vi "pmu_Check Channel Error (Std 2011).vi"(8 "error in (no error)":errorcluster, 10 "physical channel in":T3(array[cluster]), 11 "phasor channels":T4[](array[typedef]) {"phasor unit scaling" max=16777215 format="%06x"; "phasor unit" items=["Voltage [V]"=0, "Current [A]"=16777216]}) -> (0 "error out":errorcluster, 3 "phasor channel info":T1[](array[typedef]))   [LabVIEW 2014, in "NI_EP_PMU.lvlib"]
uses:
  <vilib>/addons/Electrical Power/PMU/NI_EP_PMU.lvlib
  <vilib>/addons/Electrical Power/PMU/Common/Controls/pmu_Phasor Channel.ctl
  <vilib>/addons/Electrical Power/PMU/Common/Controls/pmu_Channel Phase.ctl
  <vilib>/addons/Electrical Power/PMU/Common/Controls/pmu_Phasor Channel Info.ctl
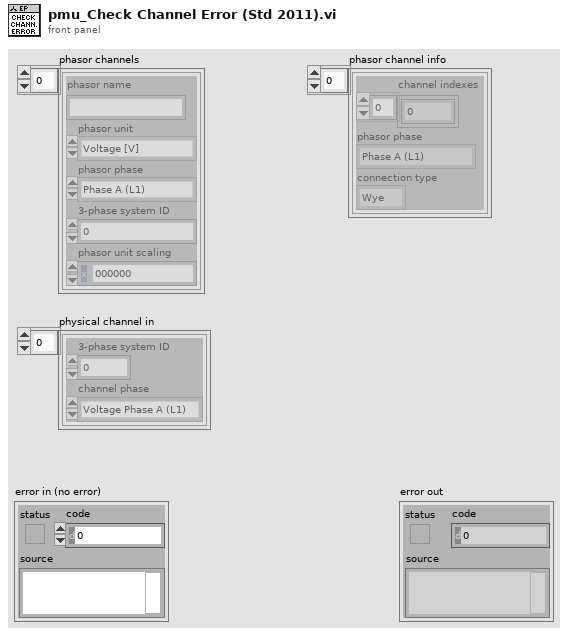
[diagram p1: front panel]
types:
  T1 = typedef "NI_EP_PMU.lvlib/pmu_Phasor Channel Info.ctl" = cluster{"channel indexes":i32[], "phasor phase":enum16{"Phase A (L1)", "Phase B (L2)", "Phase C (L3)", "Phase N", "Positive sequence", "Negative sequence", "Zero sequence"}, "connection type":enum16{"Wye", "Delta"}}
  T2 = typedef "NI_EP_PMU.lvlib/pmu_Channel Phase.ctl" = enum16{"Voltage Phase A (L1)", "Voltage Phase B (L2)", "Voltage Phase C (L3)", "Voltage Phase N (Neutral)", "Current Phase A (L1)", "Current Phase B (L2)", "Current Phase C (L3)", "Current Phase N (Neutral)", "Voltage Phase AB (L1L2)", "Voltage Phase BC (L2L3)", "Voltage Phase CA (L3L1)"}
  T3 = cluster{"3-phase system ID":u8, "channel phase":T2}[]
  T4 = typedef "NI_EP_PMU.lvlib/pmu_Phasor Channel.ctl" = cluster{"phasor name":string, "phasor unit":u32, "phasor phase":enum16{"Phase A (L1)", "Phase B (L2)", "Phase C (L3)", "Phase N", "Positive sequence", "Negative sequence", "Zero sequence"}, "3-phase system ID":u8, "phasor unit scaling":u32}
  T5 = enum16{"Phase A (L1)", "Phase B (L2)", "Phase C (L3)", "Phase N", "Positive sequence", "Negative sequence", "Zero sequence"}
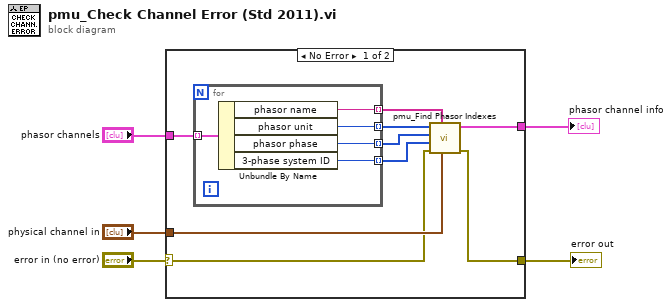
[diagram p0: block diagram]
diagram:
  n1 = case shown="No Error" "error in (no error)" {
    selector: "error in (no error)" -> [w8 w20]
    tunnel: "phasor channels" -> [w14 _]
    tunnel: "physical channel in" -> [w9 _]
    tunnel: [w6 w20] -> w1
    tunnel: [w7 _] -> w2
    frame No Error {
      n2 = for {
        tunnel: w14 -> [w19] mode=indexing
        tunnel: [w18] -> w13 mode=indexing
        tunnel: [w17] -> w12 mode=indexing
        tunnel: [w16] -> w11 mode=indexing
        tunnel: [w15] -> w10 mode=indexing
        n3 = Unbundle By Name(w19) -> ("phasor name"=w17:string, "phasor unit"=w18:u32, "phasor phase"=w16:T5, "3-phase system ID"=w15:u8)
      }
      n4 = call <vilib>:"pmu_Find Phasor Indexes.vi"("physical channel in"=w9, "phasor names"=w12, "error in (no error)"=w8, "3-phase system IDs"=w10, "phasor phases"=w11, "phasor units"=w13) -> ("error out"=w6:errorcluster, "phasor channel info"=w7:T1[])  [unwired: 4 in]
    }
    frame Error {
    }
  }
  "error out" <- w1
  "phasor channel info" <- w2
